vi "AlGaInPAs_v19.vi"(2 "Debug Mode":bool, 3 "Elapsed Time(s)":dbl, 4 "State":enum16{"Edit", "Start", "Run", "End", "Idle"}(ring), 5 "Argument List In":string[](array[string])) -> (0 "Status Out":string, 1 "Argument List Out":string[](array[string]))   [LabVIEW 2011]
panel:
  in  "As gas Active":bool
  in  "As gas main":T1 caption="Al" {"Flow" format="%.2f"}
  in  "As gas copy":cluster{}
  in  "P bubbler main":cluster{"Flow":dbl, "Run":bool, "Prep":bool} caption="Al" {"Flow" format="%.2f"}
  in  "P bubbler Active":bool
  in  "P gas copy":cluster{}
  in  "P gas Active":bool
  in  "P bubbler copy":cluster{}
  in  "P gas main":cluster{"Flow":dbl, "Run":bool, "Prep":bool} caption="Al" {"Flow" format="%.2f"}
  out "Al bubbler copy":cluster{}
  in  "Al Active":bool caption="Al bubbler Active"
  out "In bubbler copy":cluster{}
  in  "In bubbler Active":bool
  in  "In main":cluster{"Flow":dbl, "Run":bool, "Prep In":bool} caption="Al" {"Flow" format="%.2f"}
  in  "Ga bubbler Active":bool caption="Active"
  out "Ga bubbler copy":cluster{}
  in  "Al bubbler":T2 {"Panel"."Al Flow" format="%.2f"}
  out "prep_done":bool
  out "run started":bool
  out "first":bool=TRUE
  out "total time":dbl
  out "is OK?":bool
  in  "Prep In":bool caption="Pre-run"
  in  "prep_time":dbl
  in  "Cancel":bool
  in  "OK":bool
  out "tTotal(s) 2":dbl
  in  "Ga Tab Control":enum32{"Page 1", "Page 2", "Page 3"}(tab)
  in  "Ga main":T3 caption="Al" {"Flow" format="%.2f"}
  in  "MFC Flows":T4={"MFC2 flow"=10.0, "MFC3 flow"=100.0, "MFC1 flow"=1.0} {"MFC1 flow" format="%.4f"; "MFC3 flow" format="%.1f"; "MFC2 flow" format="%.2f"}
  in  "Ga Calculated":u16(ring)=1 caption="Calculated" items=["Ga flow", "MFC1", "MFC2", "MFC3"]
  # "Add pre-run time to run time in editor."
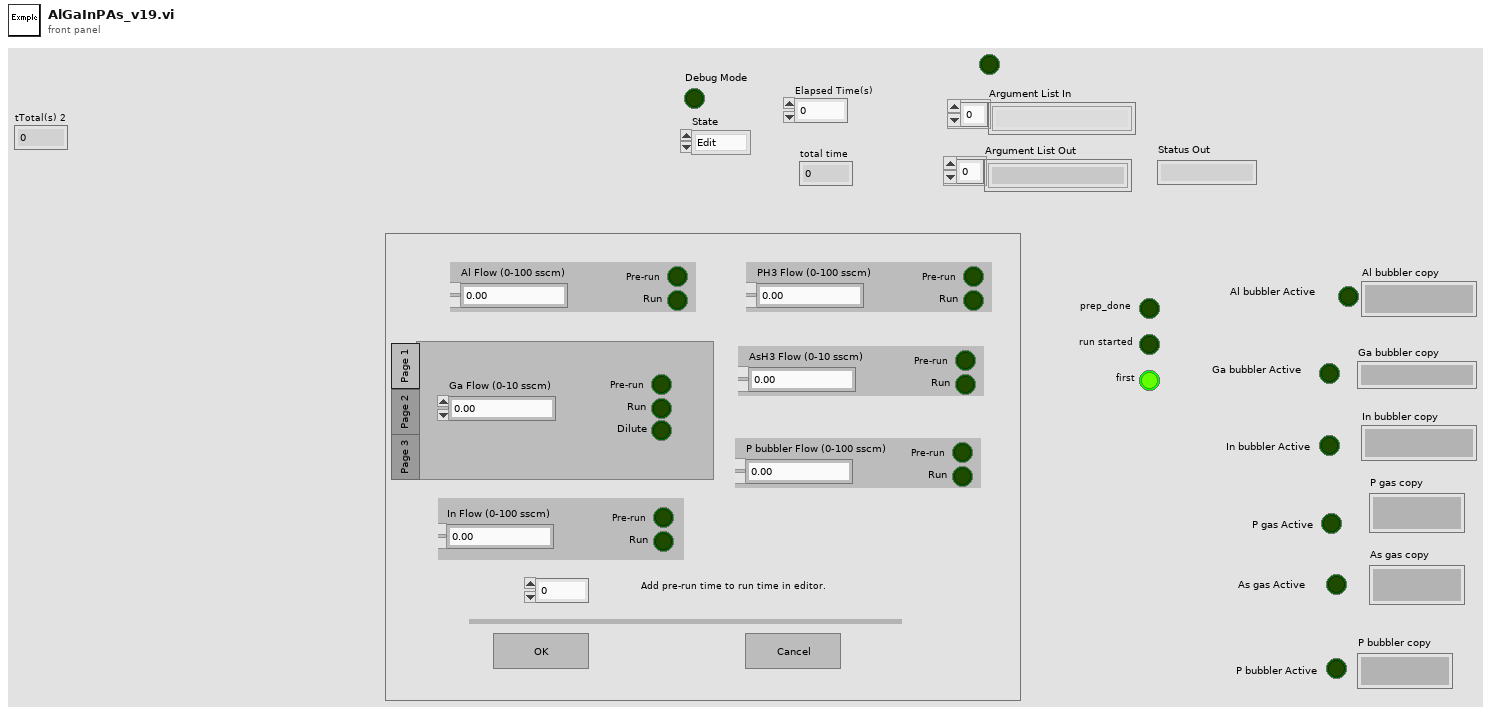
[diagram p1: front panel]
types:
  T1 = cluster{"Flow":dbl, "AsH3 Run":bool, "AsH3 Prep":bool}
  T2 = cluster{"Panel":cluster{"Al Flow":dbl, "Al Run":bool, "Prep Al":bool}}
  T3 = cluster{"Flow":dbl, "Run":bool, "Prep Ga":bool, "Dilution":bool}
  T4 = cluster{"MFC2 flow":dbl, "MFC3 flow":dbl, "MFC1 flow":dbl}
  T5 = enum16{"Discrete", "Continuous", "Instantaneous", "Finite"}
  T6 = enum32{"Invalid", "Default", "Floating", "Floating/Auto-Hide", "Modal"}
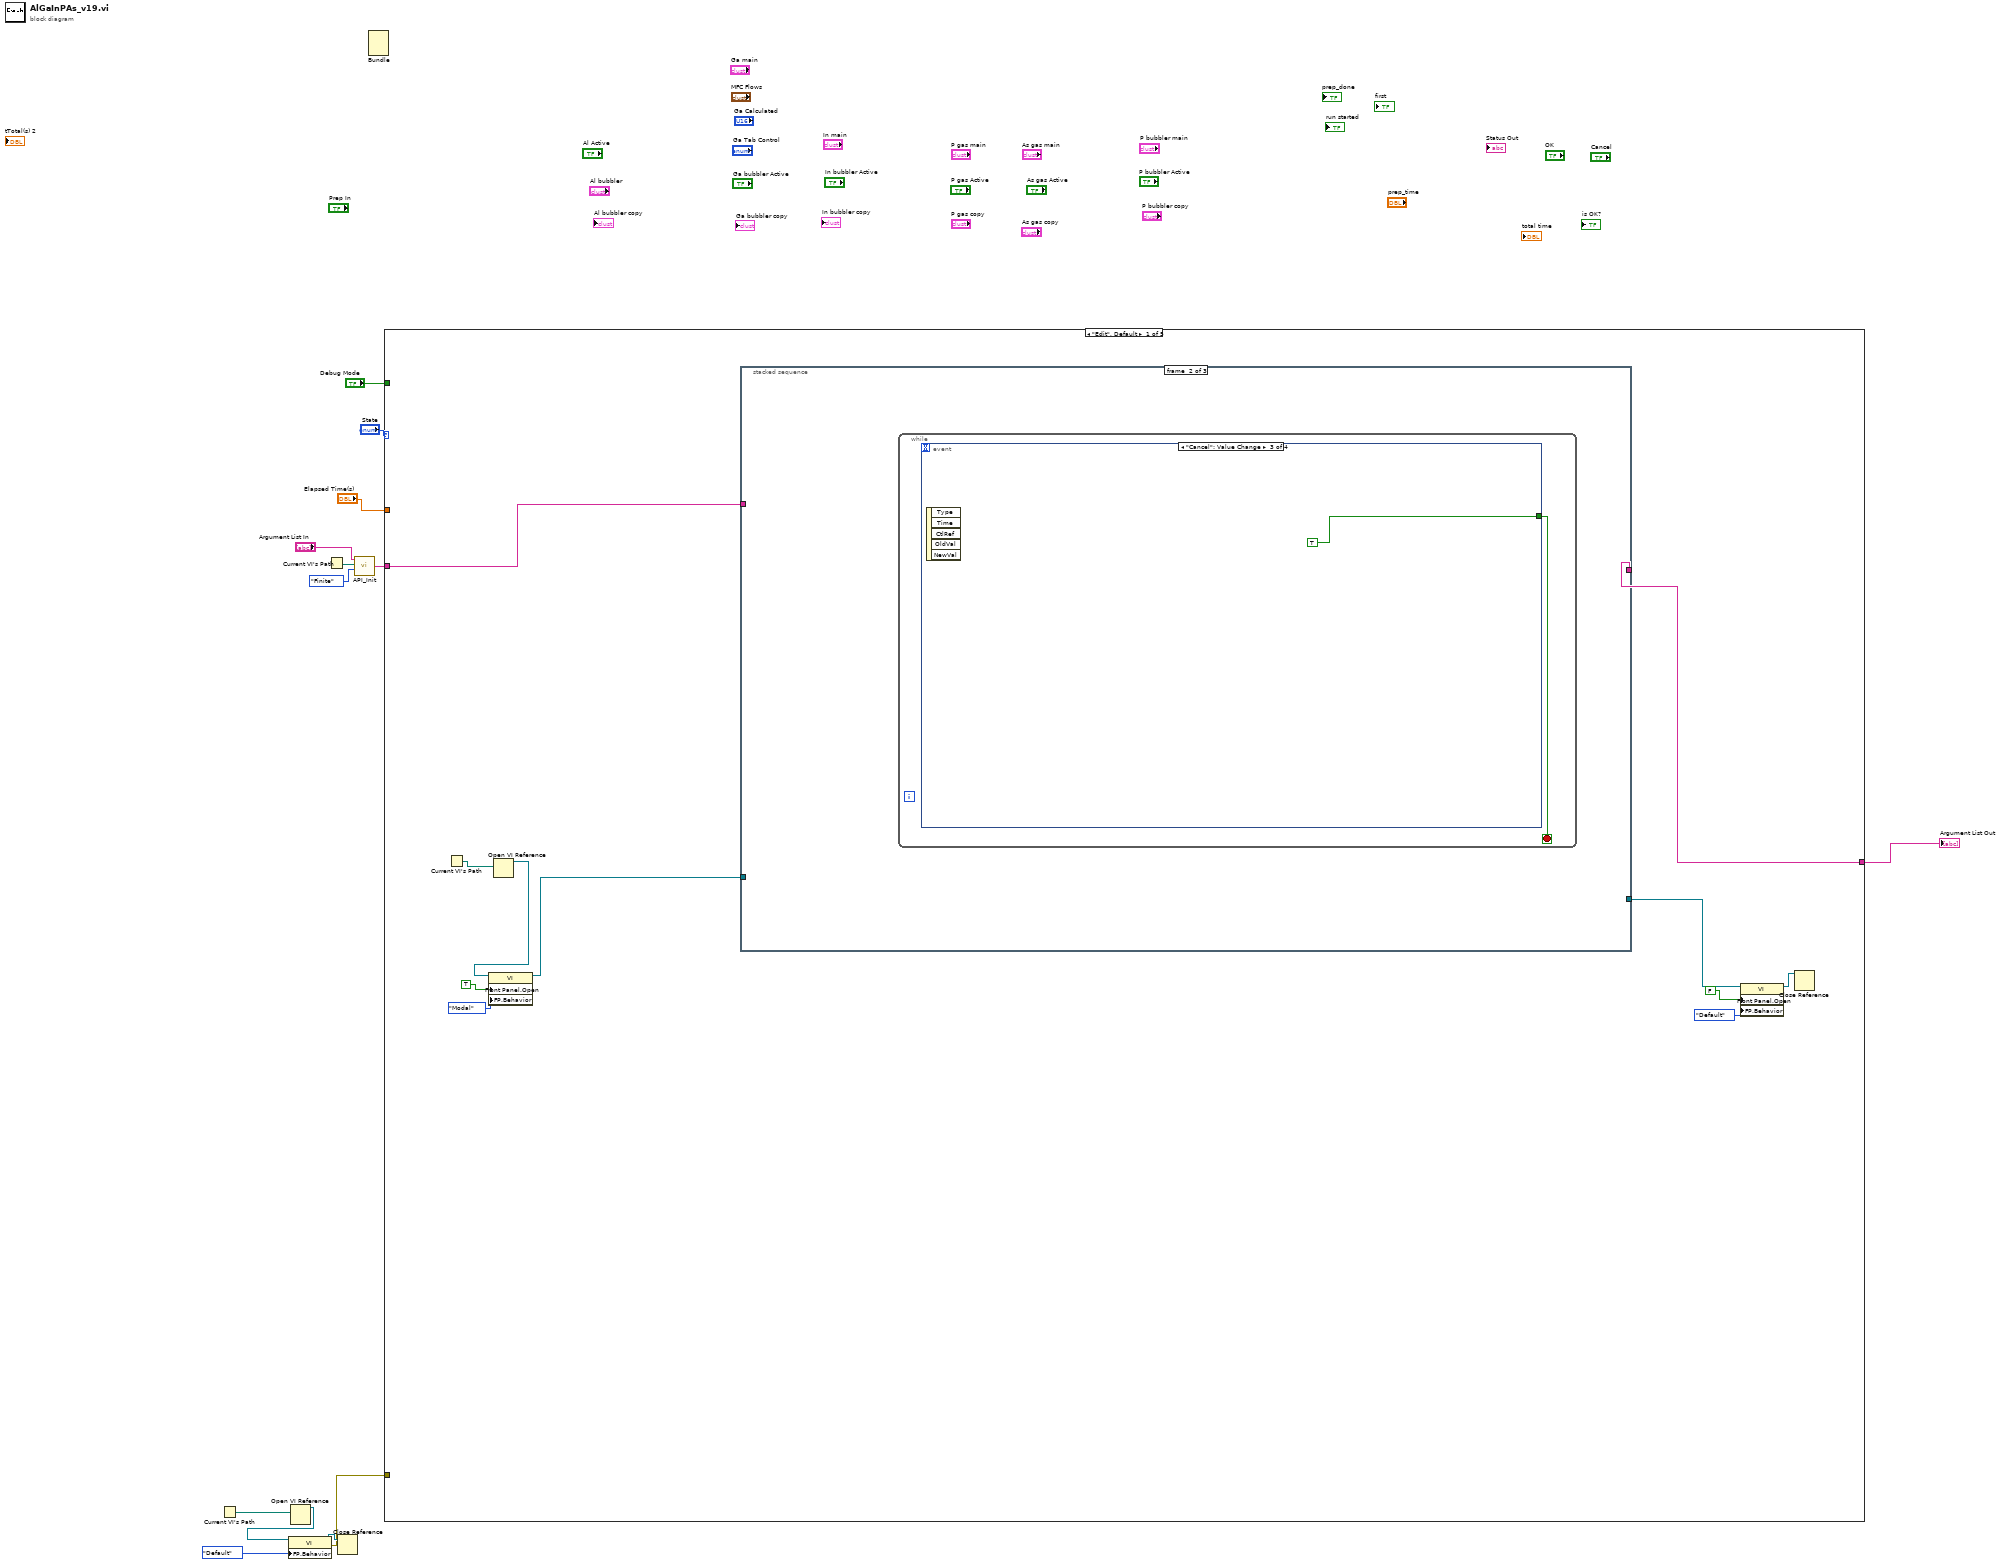
[diagram p0: block diagram]
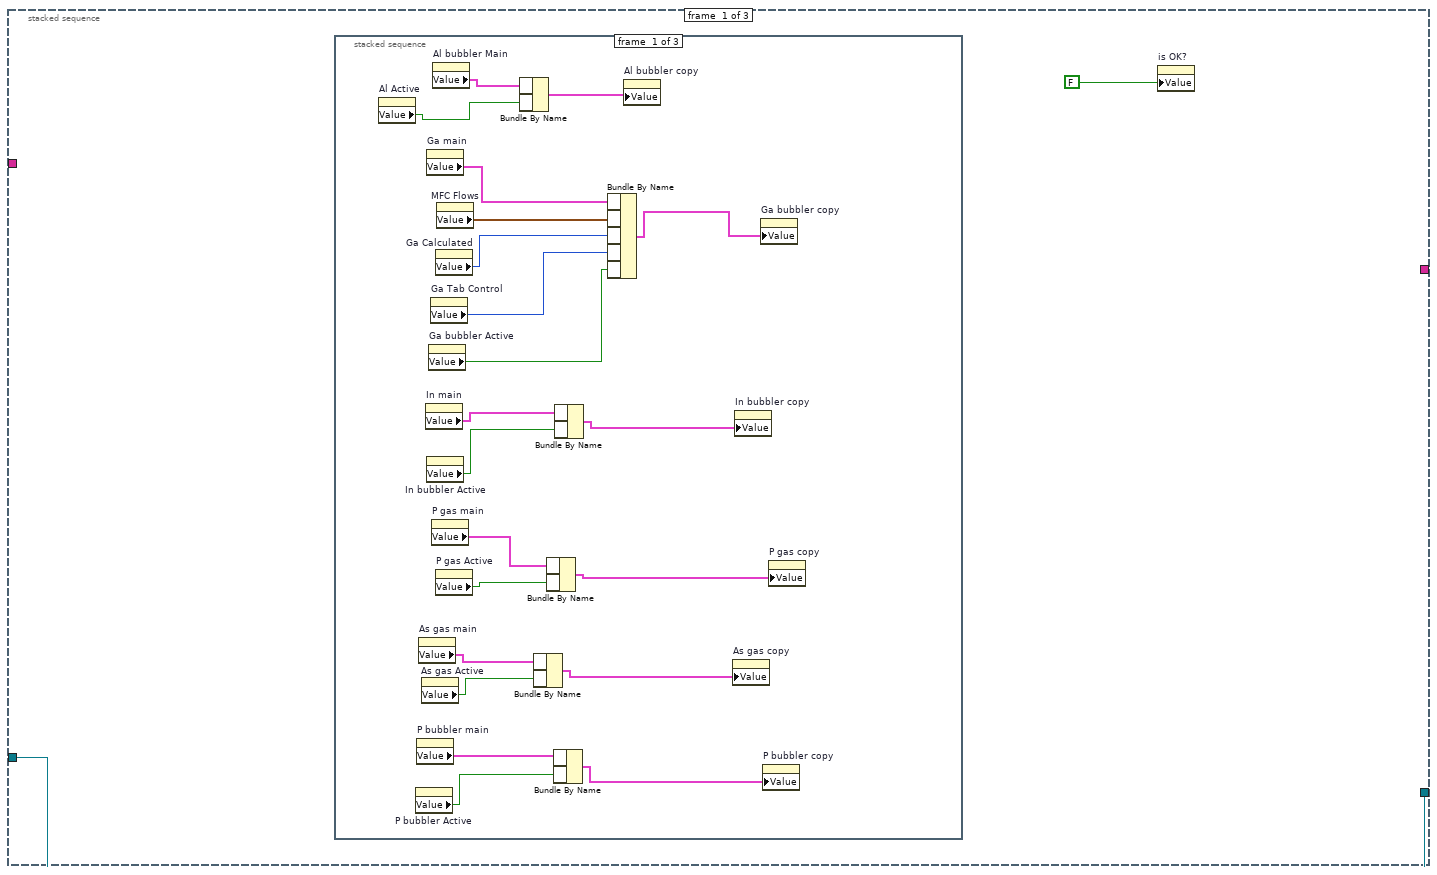
[diagram p2: hidden frame]
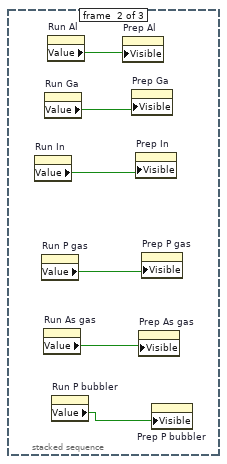
[diagram p3: hidden frame]
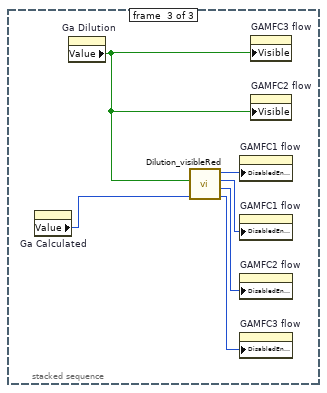
[diagram p4: hidden frame]
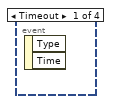
[diagram p5: hidden frame]
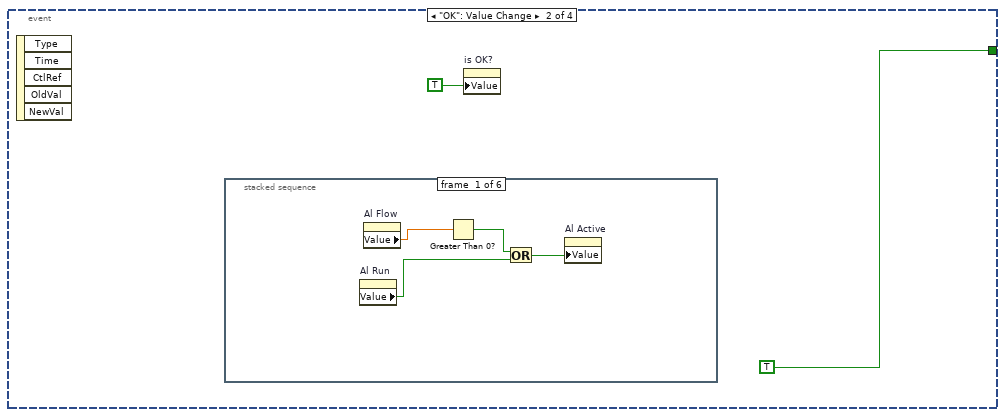
[diagram p6: hidden frame]
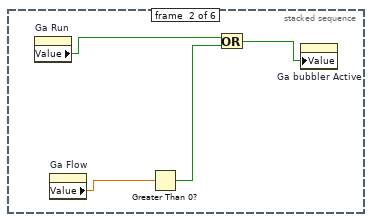
[diagram p7: hidden frame]
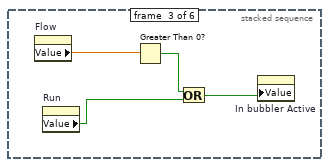
[diagram p8: hidden frame]
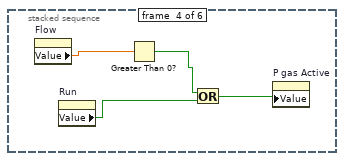
[diagram p9: hidden frame]
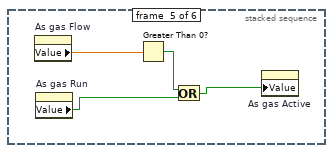
[diagram p10: hidden frame]
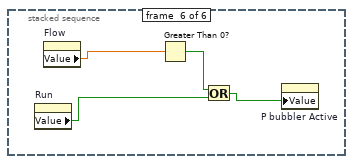
[diagram p11: hidden frame]
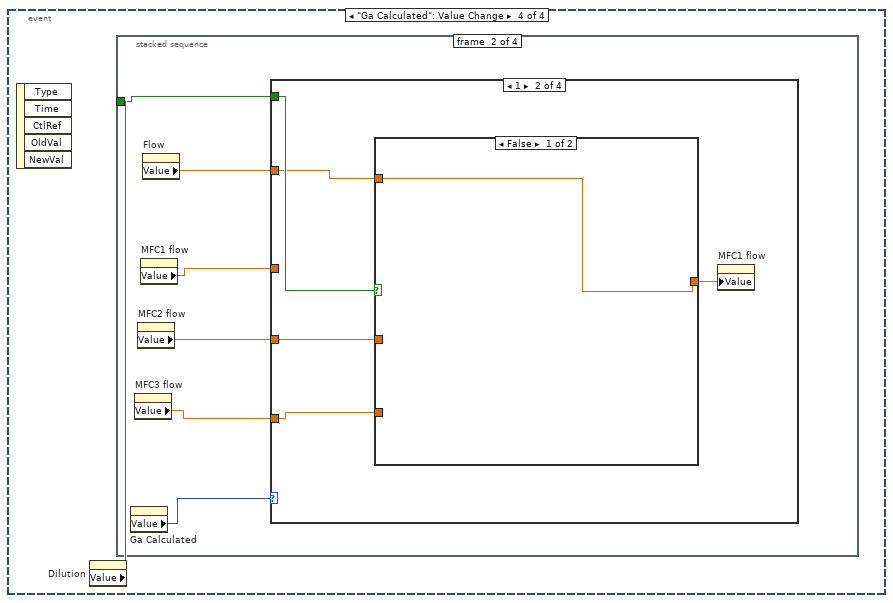
[diagram p12: hidden frame]
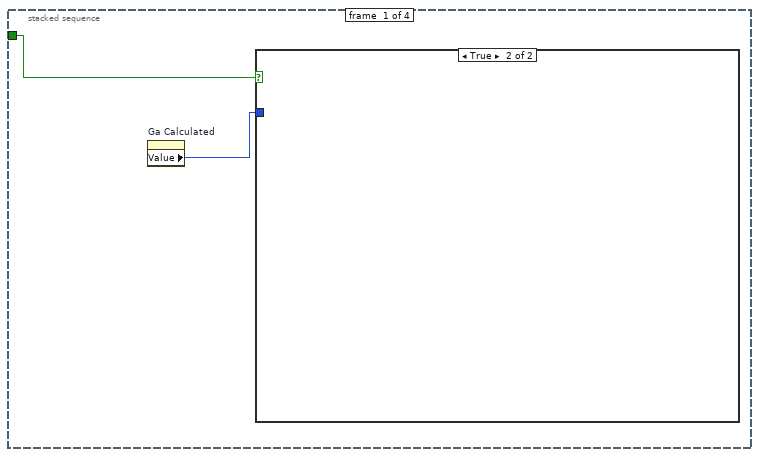
[diagram p13: hidden frame]
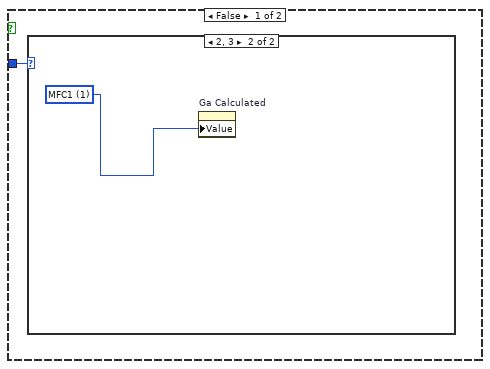
[diagram p14: hidden frame]
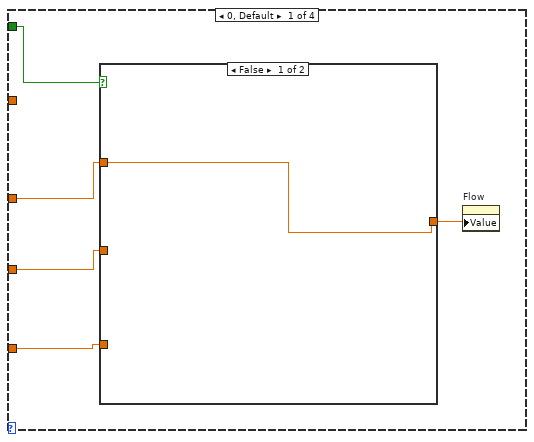
[diagram p16: hidden frame]
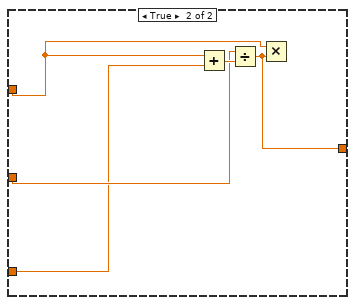
[diagram p17: hidden frame]
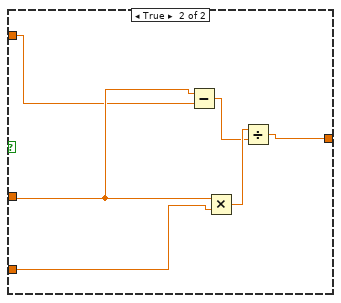
[diagram p18: hidden frame]
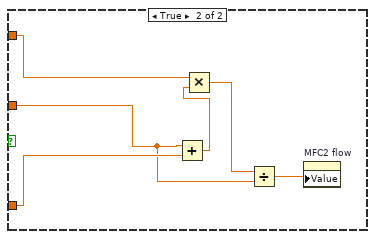
[diagram p20: hidden frame]
diagram:
  n1 = Current VI's Path() -> (path=w9:path)
  n2 = Open VI Reference(vi path=w9) -> (vi reference=w8:refnum<vi>)  [unwired: 1 in, 5 out]
  n3 = property class="VI"(reference=w8, "FP.Behavior"=T6."Default" ("Front Panel Window:Behavior")) -> (reference out=w6:refnum<vi>, error out=w5:errorcluster)  [unwired: 1 in]
  n4 = Current VI's Path() -> (path=w4:path)
  n5 = Close Reference(reference=w6) -> ()  [unwired: 1 in, 1 out]
  n6 = call "API_Init.vi"("API Mode"=T5."Finite", "VI Path"=w4, "Argument List In"="Argument List In") -> ("Argument List Out"=w1:string[])  [unwired: 1 in]
  n7 = Bundle() -> ()  [unwired: 6 in, 1 out]
  n8 = case shown="\"Edit\", Default" "State" {
    tunnel: "Debug Mode" -> [_ w159 w217 _ _]
    tunnel: "Elapsed Time(s)" -> [_ _ w218 _ _]
    tunnel: w1 -> [w15 w161 w216 w322 w323]
    tunnel: [w14 w160 w215 w322 w323] -> w10
    tunnel: w5 -> [_ _ _ _ _]
    frame "Edit", Default {
      n9 = Current VI's Path() -> (path=w20:path)
      n10 = Open VI Reference(vi path=w20) -> (vi reference=w19:refnum<vi>)  [unwired: 1 in, 5 out]
      n11 = property class="VI"(reference=w19, "Front Panel.Open"=TRUE ("Front Panel Window:Open"), "FP.Behavior"=T6."Modal" ("Front Panel Window:Behavior")) -> (reference out=w18:refnum<vi>)  [unwired: 1 in, 1 out]
      n12 = stacked-sequence {
        tunnel: w15 -> [_ _ w154]
        tunnel: w18 -> [w26 _ _]
        tunnel: [w26 _ _] -> w22
        tunnel: [_ _ w152] -> w14
        frame #0 {
          n13 = stacked-sequence {
            frame #0 {
              n14 = property on="Al Active" class="Bool (strict)"() -> ("Value"=w36:bool)  [unwired: 2 in, 2 out]
              n15 = property on="P bubbler Active" class="Bool (strict)"() -> ("Value"=w33:bool)  [unwired: 2 in, 2 out]
              n16 = property on="P bubbler main" class="Clust (strict)"() -> ("Value"=w34:cluster{"Flow":dbl, "Run":bool, "Prep":bool})  [unwired: 2 in, 2 out]
              n17 = property on="As gas main" class="Clust (strict)"() -> ("Value"=w32:T1)  [unwired: 2 in, 2 out]
              n18 = property on="As gas Active" class="Bool (strict)"() -> ("Value"=w31:bool)  [unwired: 2 in, 2 out]
              n19 = property on="In main" class="Clust (strict)"() -> ("Value"=w42:cluster{"Flow":dbl, "Run":bool, "Prep In":bool})  [unwired: 2 in, 2 out]
              n20 = property on="Ga main" class="Clust (strict)"() -> ("Value"=w39:T3)  [unwired: 2 in, 2 out]
              n21 = property on="In bubbler Active" class="Bool (strict)"() -> ("Value"=w41:bool)  [unwired: 2 in, 2 out]
              n22 = property on="Ga bubbler Active" class="Bool (strict)"() -> ("Value"=w43:bool)  [unwired: 2 in, 2 out]
              n23 = property on="Ga Tab Control" class="TabCtl (strict)"() -> ("Value"=w45:enum32{"Page 1", "Page 2", "Page 3"})  [unwired: 2 in, 2 out]
              n24 = property on="P gas main" class="Clust (strict)"() -> ("Value"=w29:cluster{"Flow":dbl, "Run":bool, "Prep":bool})  [unwired: 2 in, 2 out]
              n25 = property on="Al bubbler Main" class="Clust (strict)"() -> ("Value"=w38:T2)  [unwired: 2 in, 2 out]
              n26 = property on="Ga Calculated" class="Ring (strict)"() -> ("Value"=w46:u16)  [unwired: 2 in, 2 out]
              n27 = property on="P gas Active" class="Bool (strict)"() -> ("Value"=w28:bool)  [unwired: 2 in, 2 out]
              n28 = property on="MFC Flows" class="Clust (strict)"() -> ("Value"=w47:T4)  [unwired: 2 in, 2 out]
              n29 = Bundle By Name(w38, w36) -> (w37:cluster{})  [unwired: 1 in]
              n30 = Bundle By Name(w32, w31) -> (w30:cluster{})  [unwired: 1 in]
              n31 = Bundle By Name(w29, w28) -> (w35:cluster{})  [unwired: 1 in]
              n32 = Bundle By Name(w34, w33) -> (w27:cluster{})  [unwired: 1 in]
              n33 = Bundle By Name(w42, w41) -> (w40:cluster{})  [unwired: 1 in]
              n34 = Bundle By Name(w39, w47, w46, w45, w43) -> (w44:cluster{})  [unwired: 1 in]
              n35 = property on="Al bubbler copy" class="Clust"("Value"=w37) -> ()  [unwired: 2 in, 2 out]
              n36 = property on="As gas copy" class="Clust"("Value"=w30) -> ()  [unwired: 2 in, 2 out]
              n37 = property on="In bubbler copy" class="Clust"("Value"=w40) -> ()  [unwired: 2 in, 2 out]
              n38 = property on="Ga bubbler copy" class="Clust"("Value"=w44) -> ()  [unwired: 2 in, 2 out]
              n39 = property on="P bubbler copy" class="Clust"("Value"=w27) -> ()  [unwired: 2 in, 2 out]
              n40 = property on="P gas copy" class="Clust"("Value"=w35) -> ()  [unwired: 2 in, 2 out]
            }
            frame #1 {
              n41 = property on="Run In" class="Bool (strict)"() -> ("Value"=w52:bool)  [unwired: 2 in, 2 out]
              n42 = property on="Run P gas" class="Bool (strict)"() -> ("Value"=w50:bool)  [unwired: 2 in, 2 out]
              n43 = property on="Run As gas" class="Bool (strict)"() -> ("Value"=w49:bool)  [unwired: 2 in, 2 out]
              n44 = property on="Run Ga" class="Bool (strict)"() -> ("Value"=w51:bool)  [unwired: 2 in, 2 out]
              n45 = property on="Run Al" class="Bool (strict)"() -> ("Value"=w53:bool)  [unwired: 2 in, 2 out]
              n46 = property on="Run P bubbler" class="Bool (strict)"() -> ("Value"=w48:bool)  [unwired: 2 in, 2 out]
              n47 = property on="Prep Al" class="Bool (strict)"("Visible"=w53) -> ()  [unwired: 2 in, 2 out]
              n48 = property on="Prep Ga" class="Bool (strict)"("Visible"=w51) -> ()  [unwired: 2 in, 2 out]
              n49 = property on="Prep In" class="Bool (strict)"("Visible"=w52) -> ()  [unwired: 2 in, 2 out]
              n50 = property on="Prep As gas" class="Bool (strict)"("Visible"=w49) -> ()  [unwired: 2 in, 2 out]
              n51 = property on="Prep P gas" class="Bool (strict)"("Visible"=w50) -> ()  [unwired: 2 in, 2 out]
              n52 = property on="Prep P bubbler" class="Bool (strict)"("Visible"=w48) -> ()  [unwired: 2 in, 2 out]
            }
            frame #2 {
              n53 = property on="Ga Calculated" class="Ring (strict)"() -> ("Value"=w59:u16)  [unwired: 2 in, 2 out]
              n54 = property on="Ga Dilution" class="Bool (strict)"() -> ("Value"=w58:bool)  [unwired: 2 in, 2 out]
              n55 = call "Dilution_visibleRed.vi"("calculated"=w59, "dilution"=w58) -> ("MFC3"=w54:u16, "MFC2"=w55:u16, "MFC1"=w56:u16, "flow"=w57:u16)  [unwired: 2 in]
              n56 = property on="GAMFC1 flow" class="DigNum (strict)"("DisabledEnum"=w57) -> ()  [unwired: 2 in, 2 out]
              n57 = property on="GAMFC1 flow" class="DigNum (strict)"("DisabledEnum"=w56) -> ()  [unwired: 2 in, 2 out]
              n58 = property on="GAMFC2 flow" class="DigNum (strict)"("DisabledEnum"=w55) -> ()  [unwired: 2 in, 2 out]
              n59 = property on="GAMFC3 flow" class="DigNum (strict)"("DisabledEnum"=w54) -> ()  [unwired: 2 in, 2 out]
              n60 = property on="GAMFC3 flow" class="DigNum (strict)"("Visible"=w58) -> ()  [unwired: 2 in, 2 out]
              n61 = property on="GAMFC2 flow" class="DigNum (strict)"("Visible"=w58) -> ()  [unwired: 2 in, 2 out]
            }
          }
          n62 = property on="is OK?" class="Bool (strict)"("Value"=FALSE ("is OK?")) -> ()  [unwired: 2 in, 2 out]
        }
        frame #1 {
          n63 = while {
            stop <- w60 stop-if-true
            n64 = event shown="[2] \"Cancel\": Value Change" {
              selector: _ -> [_ _ _ _]
              dyn-events: _ -> [_ _ _ _]
              timeout: _ -> [_ _ _ _]
              tunnel: [_ TRUE TRUE _] -> w60
              event Timeout {
                n65 = event-data() -> ()  [unwired: 1 in, 2 out]
              }
              event "OK": Value Change {
                n66 = event-data() -> ()  [unwired: 1 in, 5 out]
                n67 = stacked-sequence {
                  frame #0 {
                    n68 = property on="Al Run" class="Bool (strict)"() -> ("Value"=w64:bool)  [unwired: 2 in, 2 out]
                    n69 = property on="Al Flow" class="DigNum (strict)"() -> ("Value"=w65:dbl)  [unwired: 2 in, 2 out]
                    n70 = Greater Than 0?(x=w65) -> (x > 0?=w66:bool)
                    n71 = Or(x=w66, y=w64) -> (x .or. y?=w63:bool)
                    n72 = property on="Al Active" class="Bool (strict)"("Value"=w63) -> ()  [unwired: 2 in, 2 out]
                  }
                  frame #1 {
                    n73 = property on="Ga Run" class="Bool (strict)"() -> ("Value"=w68:bool)  [unwired: 2 in, 2 out]
                    n74 = property on="Ga Flow" class="DigNum (strict)"() -> ("Value"=w67:dbl)  [unwired: 2 in, 2 out]
                    n75 = Greater Than 0?(x=w67) -> (x > 0?=w70:bool)
                    n76 = Or(x=w68, y=w70) -> (x .or. y?=w69:bool)
                    n77 = property on="Ga bubbler Active" class="Bool (strict)"("Value"=w69) -> ()  [unwired: 2 in, 2 out]
                  }
                  frame #2 {
                    n78 = property on="Flow" class="DigNum (strict)"() -> ("Value"=w73:dbl)  [unwired: 2 in, 2 out]
                    n79 = property on="Run" class="Bool (strict)"() -> ("Value"=w72:bool)  [unwired: 2 in, 2 out]
                    n80 = Greater Than 0?(x=w73) -> (x > 0?=w74:bool)
                    n81 = Or(x=w74, y=w72) -> (x .or. y?=w71:bool)
                    n82 = property on="In bubbler Active" class="Bool (strict)"("Value"=w71) -> ()  [unwired: 2 in, 2 out]
                  }
                  frame #3 {
                    n83 = property on="Flow" class="DigNum (strict)"() -> ("Value"=w77:dbl)  [unwired: 2 in, 2 out]
                    n84 = property on="Run" class="Bool (strict)"() -> ("Value"=w76:bool)  [unwired: 2 in, 2 out]
                    n85 = Greater Than 0?(x=w77) -> (x > 0?=w78:bool)
                    n86 = Or(x=w78, y=w76) -> (x .or. y?=w75:bool)
                    n87 = property on="P gas Active" class="Bool (strict)"("Value"=w75) -> ()  [unwired: 2 in, 2 out]
                  }
                  frame #4 {
                    n88 = property on="As gas Flow" class="DigNum (strict)"() -> ("Value"=w81:dbl)  [unwired: 2 in, 2 out]
                    n89 = property on="As gas Run" class="Bool (strict)"() -> ("Value"=w80:bool)  [unwired: 2 in, 2 out]
                    n90 = Greater Than 0?(x=w81) -> (x > 0?=w82:bool)
                    n91 = Or(x=w82, y=w80) -> (x .or. y?=w79:bool)
                    n92 = property on="As gas Active" class="Bool (strict)"("Value"=w79) -> ()  [unwired: 2 in, 2 out]
                  }
                  frame #5 {
                    n93 = property on="Run" class="Bool (strict)"() -> ("Value"=w84:bool)  [unwired: 2 in, 2 out]
                    n94 = property on="Flow" class="DigNum (strict)"() -> ("Value"=w85:dbl)  [unwired: 2 in, 2 out]
                    n95 = Greater Than 0?(x=w85) -> (x > 0?=w86:bool)
                    n96 = Or(x=w86, y=w84) -> (x .or. y?=w83:bool)
                    n97 = property on="P bubbler Active" class="Bool (strict)"("Value"=w83) -> ()  [unwired: 2 in, 2 out]
                  }
                }
                n98 = property on="is OK?" class="Bool (strict)"("Value"=TRUE ("is OK?")) -> ()  [unwired: 2 in, 2 out]
              }
              event "Cancel": Value Change {
                n99 = event-data() -> ()  [unwired: 1 in, 5 out]
              }
              event "Ga Calculated", "MFC Flows.MFC1 flow", "MFC Flows.MFC2 flow", "MFC Flows.MFC3 flow", "Ga main.Flow", "Ga main.Dilution": Value Change {
                n100 = event-data() -> ()  [unwired: 1 in, 5 out]
                n101 = property on="Dilution" class="Bool (strict)"() -> ("Value"=w88:bool)  [unwired: 2 in, 2 out]
                n102 = stacked-sequence {
                  tunnel: w88 -> [w89 w97 w142 w148]
                  frame #0 {
                    n103 = property on="Ga Calculated" class="Ring (strict)"() -> ("Value"=w90:u16)  [unwired: 2 in, 2 out]
                    n104 = case shown="True" w89 {
                      tunnel: w90 -> [w91 _]
                      frame False {
                        n105 = case shown="2, 3" w91 {
                          frame 0, 1, Default {
                          }
                          frame 2, 3 {
                            w92 = u16 1 items=["Ga flow", "MFC1", "MFC2", "MFC3"] ("Ga calculated")
                            n106 = property on="Ga Calculated" class="Ring (strict)"("Value"=w92) -> ()  [unwired: 2 in, 2 out]
                          }
                        }
                      }
                      frame True {
                      }
                    }
                  }
                  frame #1 {
                    n107 = property on="Ga Calculated" class="Ring (strict)"() -> ("Value"=w98:u16)  [unwired: 2 in, 2 out]
                    n108 = property on="MFC3 flow" class="DigNum (strict)"() -> ("Value"=w94:dbl)  [unwired: 2 in, 2 out]
                    n109 = property on="MFC2 flow" class="DigNum (strict)"() -> ("Value"=w95:dbl)  [unwired: 2 in, 2 out]
                    n110 = property on="MFC1 flow" class="DigNum (strict)"() -> ("Value"=w96:dbl)  [unwired: 2 in, 2 out]
                    n111 = property on="Flow" class="DigNum (strict)"() -> ("Value"=w93:dbl)  [unwired: 2 in, 2 out]
                    n112 = case shown="1" w98 {
                      tunnel: w97 -> [w103 w114 w125 w135]
                      tunnel: w96 -> [w102 _ w124 w134]
                      tunnel: w95 -> [w101 w111 _ w132]
                      tunnel: w94 -> [w100 w110 w123 _]
                      tunnel: w93 -> [_ w113 w122 w133]
                      frame 0, Default {
                        n113 = case shown="False" w103 {
                          tunnel: w102 -> [w104 w108]
                          tunnel: w101 -> [_ w107]
                          tunnel: w100 -> [_ w106]
                          tunnel: [w104 w105] -> w99
                          frame False {
                          }
                          frame True {
                            n114 = Add(x=w108, y=w106) -> (x+y=w109:dbl)
                            n115 = Divide(x=w107, y=w109) -> (x/y=w105:dbl)
                            n116 = Multiply(x=w108, y=w105) -> ()  [unwired: 1 out]
                          }
                        }
                        n117 = property on="Flow" class="DigNum (strict)"("Value"=w99) -> ()  [unwired: 2 in, 2 out]
                      }
                      frame 1 {
                        n118 = case shown="False" w114 {
                          tunnel: w113 -> [w115 w117]
                          tunnel: [w115 w116] -> w112
                          tunnel: w111 -> [_ w119]
                          tunnel: w110 -> [_ w118]
                          frame False {
                          }
                          frame True {
                            n119 = Subtract(x=w119, y=w117) -> (x-y=w120:dbl)
                            n120 = Multiply(x=w119, y=w118) -> (x*y=w121:dbl)
                            n121 = Divide(x=w121, y=w120) -> (x/y=w116:dbl)
                          }
                        }
                        n122 = property on="MFC1 flow" class="DigNum (strict)"("Value"=w112) -> ()  [unwired: 2 in, 2 out]
                      }
                      frame 2 {
                        n123 = case shown="False" w125 {
                          tunnel: w124 -> [_ w127]
                          tunnel: w123 -> [_ w129]
                          tunnel: w122 -> [_ w128]
                          frame False {
                          }
                          frame True {
                            n124 = Add(x=w127, y=w129) -> (x+y=w131:dbl)
                            n125 = Multiply(x=w128, y=w131) -> (x*y=w130:dbl)
                            n126 = Divide(x=w130, y=w127) -> (x/y=w126:dbl)
                            n127 = property on="MFC2 flow" class="DigNum (strict)"("Value"=w126) -> ()  [unwired: 2 in, 2 out]
                          }
                        }
                      }
                      frame 3 {
                        n128 = case shown="False" w135 {
                          tunnel: w134 -> [_ w139]
                          tunnel: w133 -> [_ w138]
                          tunnel: w132 -> [_ w137]
                          frame False {
                          }
                          frame True {
                            n129 = Subtract(x=w137, y=w138) -> (x-y=w140:dbl)
                            n130 = Divide(x=w139, y=w138) -> (x/y=w141:dbl)
                            n131 = Multiply(x=w141, y=w140) -> (x*y=w136:dbl)
                            n132 = property on="MFC3 flow" class="DigNum (strict)"("Value"=w136) -> ()  [unwired: 2 in, 2 out]
                          }
                        }
                      }
                    }
                  }
                  frame #2 {
                    n133 = property on="Ga Calculated" class="Ring (strict)"() -> ("Value"=w147:u16)  [unwired: 2 in, 2 out]
                    n134 = call "Dilution_visibleRed.vi"("calculated"=w147, "dilution"=w142) -> ("MFC3"=w143:u16, "MFC2"=w144:u16, "MFC1"=w145:u16, "flow"=w146:u16)  [unwired: 2 in]
                    n135 = property on="MFC3 flow" class="DigNum (strict)"("Visible"=w142) -> ()  [unwired: 2 in, 2 out]
                    n136 = property on="Flow" class="DigNum (strict)"("DisabledEnum"=w146) -> ()  [unwired: 2 in, 2 out]
                    n137 = property on="MFC3 flow" class="DigNum (strict)"("DisabledEnum"=w143) -> ()  [unwired: 2 in, 2 out]
                    n138 = property on="MFC2 flow" class="DigNum (strict)"("Visible"=w142) -> ()  [unwired: 2 in, 2 out]
                    n139 = property on="MFC2 flow" class="DigNum (strict)"("DisabledEnum"=w144) -> ()  [unwired: 2 in, 2 out]
                    n140 = property on="MFC1 flow" class="DigNum (strict)"("DisabledEnum"=w145) -> ()  [unwired: 2 in, 2 out]
                  }
                  frame #3 {
                    n141 = case shown="True" w148 {
                      frame False {
                        n142 = property on="Ga Calculated" class="Ring (strict)"("Disabled Items []"=i32[] [2, 3]) -> ()  [unwired: 2 in, 2 out]
                      }
                      frame True {
                        n143 = property on="Ga Calculated" class="Ring (strict)"("Disabled Items []"=i32[] []) -> ()  [unwired: 2 in, 2 out]
                      }
                    }
                  }
                }
              }
            }
          }
        }
        frame #2 {
          n144 = property on="is OK?" class="Bool (strict)"() -> ("Value"=w151:bool)  [unwired: 2 in, 2 out]
          n145 = case shown="True" w151 {
            tunnel: w154 -> [w157 w158]
            tunnel: [w157 w158] -> w153
            frame False {
            }
            frame True {
            }
          }
          n146 = Not(x=w151) -> (.not. x?=w156:bool)
          n147 = Current VI's Path() -> (path=w155:path)
          n148 = call "API_Edit.vi"("Cancel"=w156, "OK"=w151, "VI Path"=w155, "Argument List In"=w153) -> ("Argument List Out"=w152:string[])
        }
      }
      n149 = property class="VI"(reference=w22, "Front Panel.Open"=FALSE ("Front Panel Window:Open"), "FP.Behavior"=T6."Default" ("Front Panel Window:Behavior")) -> (reference out=w23:refnum<vi>)  [unwired: 1 in, 1 out]
      n150 = Close Reference(reference=w23) -> ()  [unwired: 1 in, 1 out]
    }
    frame "Start" {
      n151 = call "Set_Argument.vi"("Enable"=FALSE, "Argument"="run_started", "Argument List In"=w161) -> ("Argument List Out"=w160:string[])
      n152 = case shown="False" w159 {
        frame False {
          n153 = stacked-sequence {
            frame #0 {
              n154 = property on="Al Active" class="Bool (strict)"() -> ("Value"=w164:bool)  [unwired: 2 in, 2 out]
              n155 = case shown="False" w164 {
                frame False {
                  w165 = FALSE ("Al Active")
                  n156 = call "set_Al.vi"("ALMFC1"=0.0 ("Aluminum Flow"), "Remote"=w165, "Run"=w165, "Bubbler In"=w165, "Active"=w165) -> ()  [unwired: 5 out]
                }
                frame True {
                  w171 = TRUE ("Al Active")
                  n157 = property on="Al Run" class="Bool (strict)"() -> ("Value"=w167:bool)  [unwired: 2 in, 2 out]
                  n158 = property on="Prep Al" class="Bool (strict)"() -> ("Value"=w168:bool)  [unwired: 2 in, 2 out]
                  n159 = And(x=w168, y=w167) -> (x .and. y?=w170:bool)
                  n160 = property on="Al Flow" class="DigNum (strict)"() -> ("Value"=w169:dbl)  [unwired: 2 in, 2 out]
                  n161 = call "set_Al.vi"("ALMFC1"=w169, "Run"=w170, "Bubbler In"=w171, "Active"=w171) -> ()  [unwired: 1 in, 5 out]
                }
              }
            }
            frame #1 {
              n162 = property on="Ga bubbler Active" class="Bool (strict)"() -> ("Value"=w172:bool)  [unwired: 2 in, 2 out]
              n163 = case shown="True" w172 {
                frame False {
                  w174 = FALSE ("Ga Active")
                  w173 = 0.0 ("Ga Flow 1")
                  n164 = call "set_Ga.vi"("Active"=w174, "GAMFC3"=w173, "GAMFC2"=w173, "GAMFC1"=w173, "Bubbler In"=w174, "H2 Dilute"=w174, "Run"=w174, "Remote"=w174) -> ()  [unwired: 8 out]
                }
                frame True {
                  w181 = TRUE ("Ga Active")
                  n165 = property on="Prep Ga" class="Bool (strict)"() -> ("Value"=w178:bool)  [unwired: 2 in, 2 out]
                  n166 = property on="Dilution" class="Bool (strict)"() -> ("Value"=w180:bool)  [unwired: 2 in, 2 out]
                  n167 = property on="MFC1 flow" class="DigNum (strict)"() -> ("Value"=w177:dbl)  [unwired: 2 in, 2 out]
                  n168 = property on="Run" class="Bool (strict)"() -> ("Value"=w179:bool)  [unwired: 2 in, 2 out]
                  n169 = And(x=w178, y=w179) -> (x .and. y?=w182:bool)
                  n170 = property on="MFC2 flow" class="DigNum (strict)"() -> ("Value"=w176:dbl)  [unwired: 2 in, 2 out]
                  n171 = property on="MFC3 flow" class="DigNum (strict)"() -> ("Value"=w175:dbl)  [unwired: 2 in, 2 out]
                  n172 = call "set_Ga.vi"("Active"=w181, "GAMFC3"=w175, "GAMFC2"=w176, "GAMFC1"=w177, "Bubbler In"=w181, "H2 Dilute"=w180, "Run"=w182, "Remote"=w181) -> ()  [unwired: 8 in]
                }
              }
            }
            frame #2 {
              n173 = property on="In bubbler Active" class="Bool (strict)"() -> ("Value"=w183:bool)  [unwired: 2 in, 2 out]
              n174 = case shown="False" w183 {
                frame False {
                  w185 = FALSE ("In Remote")
                  n175 = call "set_In.vi"("INMFC1"=0.0 ("Indium Flow"), "Remote"=w185, "Run"=w185, "Bubbler In"=w185, "Active"=w185) -> ()  [unwired: 5 out]
                }
                frame True {
                  w190 = TRUE ("In Run")
                  n176 = property on="Run" class="Bool (strict)"() -> ("Value"=w187:bool)  [unwired: 2 in, 2 out]
                  n177 = property on="Prep In" class="Bool (strict)"() -> ("Value"=w188:bool)  [unwired: 2 in, 2 out]
                  n178 = And(x=w187, y=w188) -> (x .and. y?=w189:bool)
                  n179 = property on="Flow" class="DigNum (strict)"() -> ("Value"=w186:dbl)  [unwired: 2 in, 2 out]
                  n180 = call "set_In.vi"("INMFC1"=w186, "Run"=w189, "Bubbler In"=w190, "Active"=w190) -> ()  [unwired: 1 in, 5 out]
                }
              }
            }
            frame #3 {
              n181 = property on="P gas Active" class="Bool (strict)"() -> ("Value"=w191:bool)  [unwired: 2 in, 2 out]
              n182 = case shown="False" w191 {
                frame False {
                  w192 = FALSE ("P_Gas Active")
                  n183 = call "set_P_gas.vi"("Run"=w192, "Gas In"=w192, "Active"=w192, "P_Gas Remote"=w192, "H2 Flush"=w192, "P_Gas Flow"=0.0) -> ()
                }
                frame True {
                  w198 = TRUE ("P_Gas Active")
                  n184 = property on="Flow" class="DigNum (strict)"() -> ("Value"=w196:dbl)  [unwired: 2 in, 2 out]
                  n185 = property on="Prep" class="Bool (strict)"() -> ("Value"=w195:bool)  [unwired: 2 in, 2 out]
                  n186 = property on="Run" class="Bool (strict)"() -> ("Value"=w194:bool)  [unwired: 2 in, 2 out]
                  n187 = And(x=w195, y=w194) -> (x .and. y?=w197:bool)
                  n188 = call "set_P_gas.vi"("Active"=w198, "P_Gas Remote"=w197, "H2 Flush"=w198, "P_Gas Flow"=w196) -> ()  [unwired: 2 in]
                }
              }
            }
            frame #4 {
              n189 = property on="As gas Active" class="Bool (strict)"() -> ("Value"=w199:bool)  [unwired: 2 in, 2 out]
              n190 = case shown="False" w199 {
                frame False {
                  w200 = FALSE ("As_Gas Active")
                  n191 = call "set_As_gas.vi"("Active"=w200, "As_Gas Flow"=0.0, "Gas In"=w200, "H2 Flush"=w200, "Run"=w200, "Remote"=w200) -> ()  [unwired: 10 in]
                }
                frame True {
                  w206 = TRUE ("As_Gas Active")
                  n192 = property on="AsH3 Run" class="Bool (strict)"() -> ("Value"=w202:bool)  [unwired: 2 in, 2 out]
                  n193 = property on="AsH3 Prep" class="Bool (strict)"() -> ("Value"=w203:bool)  [unwired: 2 in, 2 out]
                  n194 = And(x=w203, y=w202) -> (x .and. y?=w205:bool)
                  n195 = property on="Flow" class="DigNum (strict)"() -> ("Value"=w204:dbl)  [unwired: 2 in, 2 out]
                  n196 = call "set_As_gas.vi"("Active"=w206, "As_Gas Flow"=w204, "Gas In"=w206, "Run"=w205) -> ()  [unwired: 12 in]
                }
              }
            }
            frame #5 {
              n197 = property on="P bubbler Active" class="Bool (strict)"() -> ("Value"=w207:bool)  [unwired: 2 in, 2 out]
              n198 = case shown="False" w207 {
                frame False {
                  w208 = FALSE ("As_Gas Active")
                  n199 = call "set_P_Liq.vi"("flow 1"=0.0 ("As_Gas Flow"), "Remote"=w208, "Run"=w208, "Bubbler In"=w208, "Active"=w208) -> ()  [unwired: 5 in]
                }
                frame True {
                  w214 = TRUE ("As_Gas Active")
                  n200 = property on="Run" class="Bool (strict)"() -> ("Value"=w210:bool)  [unwired: 2 in, 2 out]
                  n201 = property on="Prep" class="Bool (strict)"() -> ("Value"=w211:bool)  [unwired: 2 in, 2 out]
                  n202 = And(x=w211, y=w210) -> (x .and. y?=w213:bool)
                  n203 = property on="Flow" class="DigNum (strict)"() -> ("Value"=w212:dbl)  [unwired: 2 in, 2 out]
                  n204 = call "set_P_Liq.vi"("flow 1"=w212, "Run"=w213, "Bubbler In"=w214, "Active"=w214) -> ()  [unwired: 6 in]
                }
              }
            }
          }
        }
        frame True {
        }
      }
    }
    frame "Run" {
      n205 = stacked-sequence {
        tunnel: w218 -> [_ w223 _ _]
        tunnel: w216 -> [w220 _ _ w275]
        tunnel: w217 -> [_ _ _ w274]
        tunnel: [_ _ _ w268] -> w215
        frame #0 {
          n206 = call "Get_Argument.vi"("Argument"="run_started", "Argument List"=w220) -> ("Enabled"=w219:bool)
          n207 = local write "run started"(w219) -> ()
        }
        frame #1 {
          n208 = property on="prep_time" class="DigNum (strict)"() -> ("Value"=w224:dbl)  [unwired: 2 in, 2 out]
          n209 = Greater Or Equal?(x=w223, y=w224) -> (x >= y?=w222:bool)
          n210 = local write "prep_done"(w222) -> ()
        }
        frame #2 {
          n211 = local read "run started"() -> (w226:bool)
          n212 = Not(x=w226) -> (.not. x?=w225:bool)
          n213 = stacked-sequence {
            tunnel: w225 -> [w228 w231 w237 w243 w250 w256 w262]
            frame #0 {
              n214 = case shown="True" w228 {
                tunnel: ["run: " "pre-run: "] -> w227
                frame False {
                }
                frame True {
                }
              }
              n215 = property on="Status Out" class="Str"("Value"=w227) -> ()  [unwired: 2 in, 2 out]
            }
            frame #1 {
              n216 = property on="Status Out" class="Str"() -> ("Value"=w236:string)  [unwired: 2 in, 2 out]
              n217 = call "flow_strings.vi"("string in"=w236, "is first in?"=TRUE, "name"="Al", "is prep?"=w231) -> ("string out"=w235:string, "is first out?"=w234:bool)  [unwired: 3 in]
              n218 = property on="Status Out" class="Str"("Value"=w235) -> ()  [unwired: 2 in, 2 out]
              n219 = property on="first" class="Bool (strict)"("Value"=w234) -> ()  [unwired: 2 in, 2 out]
            }
            frame #2 {
              n220 = property on="first" class="Bool (strict)"() -> ("Value"=w239:bool)  [unwired: 2 in, 2 out]
              n221 = property on="Status Out" class="Str"() -> ("Value"=w241:string)  [unwired: 2 in, 2 out]
              n222 = call "flow_strings.vi"("string in"=w241, "is first in?"=w239, "name"="Ga", "is prep?"=w237) -> ("string out"=w242:string, "is first out?"=w238:bool)  [unwired: 3 in]
              n223 = property on="Status Out" class="Str"("Value"=w242) -> ()  [unwired: 2 in, 2 out]
              n224 = property on="first" class="Bool (strict)"("Value"=w238) -> ()  [unwired: 2 in, 2 out]
            }
            frame #3 {
              n225 = property on="first" class="Bool (strict)"() -> ("Value"=w247:bool)  [unwired: 2 in, 2 out]
              n226 = property on="Status Out" class="Str"() -> ("Value"=w249:string)  [unwired: 2 in, 2 out]
              n227 = property on="Prep In" class="Bool (strict)"() -> ("Value"=w244:bool)  [unwired: 2 in, 2 out]
              n228 = call "flow_strings.vi"("string in"=w249, "is first in?"=w247, "name"="In", "prep source?"=w244, "is prep?"=w243) -> ("string out"=w246:string, "is first out?"=w245:bool)  [unwired: 2 in]
              n229 = property on="Status Out" class="Str"("Value"=w246) -> ()  [unwired: 2 in, 2 out]
              n230 = property on="first" class="Bool (strict)"("Value"=w245) -> ()  [unwired: 2 in, 2 out]
            }
            frame #4 {
              n231 = property on="first" class="Bool (strict)"() -> ("Value"=w252:bool)  [unwired: 2 in, 2 out]
              n232 = property on="Status Out" class="Str"() -> ("Value"=w254:string)  [unwired: 2 in, 2 out]
              n233 = call "flow_strings.vi"("string in"=w254, "is first in?"=w252, "name"="PH3", "is prep?"=w250) -> ("string out"=w253:string, "is first out?"=w251:bool)  [unwired: 3 in]
              n234 = property on="Status Out" class="Str"("Value"=w253) -> ()  [unwired: 2 in, 2 out]
              n235 = property on="first" class="Bool (strict)"("Value"=w251) -> ()  [unwired: 2 in, 2 out]
            }
            frame #5 {
              n236 = property on="first" class="Bool (strict)"() -> ("Value"=w258:bool)  [unwired: 2 in, 2 out]
              n237 = property on="Status Out" class="Str"() -> ("Value"=w260:string)  [unwired: 2 in, 2 out]
              n238 = call "flow_strings.vi"("string in"=w260, "is first in?"=w258, "name"="AsH3", "is prep?"=w256) -> ("string out"=w257:string, "is first out?"=w259:bool)  [unwired: 3 in]
              n239 = property on="Status Out" class="Str"("Value"=w257) -> ()  [unwired: 2 in, 2 out]
              n240 = property on="first" class="Bool (strict)"("Value"=w259) -> ()  [unwired: 2 in, 2 out]
            }
            frame #6 {
              n241 = property on="first" class="Bool (strict)"() -> ("Value"=w265:bool)  [unwired: 2 in, 2 out]
              n242 = property on="Status Out" class="Str"() -> ("Value"=w267:string)  [unwired: 2 in, 2 out]
              n243 = call "flow_strings.vi"("string in"=w267, "is first in?"=w265, "name"="P liq", "is prep?"=w262) -> ("string out"=w264:string, "is first out?"=w263:bool)  [unwired: 3 in]
              n244 = property on="Status Out" class="Str"("Value"=w264) -> ()  [unwired: 2 in, 2 out]
              n245 = property on="first" class="Bool (strict)"("Value"=w263) -> ()  [unwired: 2 in, 2 out]
            }
          }
        }
        frame #3 {
          n246 = local read "prep_done"() -> (w272:bool)
          n247 = local read "run started"() -> (w271:bool)
          n248 = Not(x=w272) -> (.not. x?=w270:bool)
          n249 = Or(x=w270, y=w271) -> (x .or. y?=w269:bool)
          n250 = Or(x=w274, y=w269) -> (x .or. y?=w273:bool)
          n251 = case shown="False" w273 {
            tunnel: w275 -> [w277 _]
            tunnel: [w276 _] -> w268
            frame False {
              n252 = stacked-sequence {
                tunnel: [_ _ _ _ _ _ w319] -> w276
                tunnel: w277 -> [_ _ _ _ _ _ w318]
                frame #0 {
                  n253 = property on="Al Active" class="Bool (strict)"() -> ("Value"=w278:bool)  [unwired: 2 in, 2 out]
                  n254 = case shown="True" w278 {
                    frame False {
                      w279 = FALSE ("Al Active")
                      n255 = call "set_Al.vi"("ALMFC1"=0.0 ("Aluminum Flow"), "Remote"=w279, "Run"=w279, "Bubbler In"=w279, "Active"=w279) -> ()  [unwired: 5 out]
                    }
                    frame True {
                      w283 = TRUE ("Al Active")
                      n256 = property on="Al Flow" class="DigNum (strict)"() -> ("Value"=w282:dbl)  [unwired: 2 in, 2 out]
                      n257 = property on="Al Run" class="Bool (strict)"() -> ("Value"=w281:bool)  [unwired: 2 in, 2 out]
                      n258 = call "set_Al.vi"("ALMFC1"=w282, "Run"=w281, "Bubbler In"=w283, "Active"=w283) -> ()  [unwired: 1 in, 5 out]
                    }
                  }
                }
                frame #1 {
                  n259 = property on="Ga bubbler Active" class="Bool (strict)"() -> ("Value"=w284:bool)  [unwired: 2 in, 2 out]
                  n260 = case shown="False" w284 {
                    frame False {
                      w286 = FALSE ("Ga Active")
                      w285 = 0.0 ("Ga Flow 1")
                      n261 = call "set_Ga.vi"("Active"=w286, "GAMFC3"=w285, "GAMFC2"=w285, "GAMFC1"=w285, "Bubbler In"=w286, "H2 Dilute"=w286, "Run"=w286, "Remote"=w286) -> ()  [unwired: 8 out]
                    }
                    frame True {
                      w292 = TRUE ("Ga Active")
                      n262 = property on="MFC2 flow" class="DigNum (strict)"() -> ("Value"=w288:dbl)  [unwired: 2 in, 2 out]
                      n263 = property on="MFC3 flow" class="DigNum (strict)"() -> ("Value"=w287:dbl)  [unwired: 2 in, 2 out]
                      n264 = property on="Run" class="Bool (strict)"() -> ("Value"=w291:bool)  [unwired: 2 in, 2 out]
                      n265 = property on="MFC1 flow" class="DigNum (strict)"() -> ("Value"=w289:dbl)  [unwired: 2 in, 2 out]
                      n266 = property on="Dilution" class="Bool (strict)"() -> ("Value"=w290:bool)  [unwired: 2 in, 2 out]
                      n267 = call "set_Ga.vi"("Active"=w292, "GAMFC3"=w287, "GAMFC2"=w288, "GAMFC1"=w289, "Bubbler In"=w292, "H2 Dilute"=w290, "Run"=w291, "Remote"=w292) -> ()  [unwired: 8 in]
                    }
                  }
                }
                frame #2 {
                  n268 = property on="In bubbler Active" class="Bool (strict)"() -> ("Value"=w293:bool)  [unwired: 2 in, 2 out]
                  n269 = case shown="True" w293 {
                    frame False {
                      w295 = FALSE ("In Remote")
                      n270 = call "set_In.vi"("INMFC1"=0.0 ("Indium Flow"), "Remote"=w295, "Run"=w295, "Bubbler In"=w295, "Active"=w295) -> ()  [unwired: 5 out]
                    }
                    frame True {
                      w298 = TRUE ("In Run")
                      n271 = property on="Run" class="Bool (strict)"() -> ("Value"=w296:bool)  [unwired: 2 in, 2 out]
                      n272 = property on="In Flow" class="DigNum (strict)"() -> ("Value"=w297:dbl)  [unwired: 2 in, 2 out]
                      n273 = call "set_In.vi"("INMFC1"=w297, "Run"=w296, "Bubbler In"=w298, "Active"=w298) -> ()  [unwired: 1 in, 5 out]
                    }
                  }
                }
                frame #3 {
                  n274 = property on="P gas Active" class="Bool (strict)"() -> ("Value"=w299:bool)  [unwired: 2 in, 2 out]
                  n275 = case shown="False" w299 {
                    frame False {
                      w300 = FALSE ("P_Gas Active")
                      n276 = call "set_P_gas.vi"("Run"=w300, "Gas In"=w300, "Active"=w300, "P_Gas Remote"=w300, "H2 Flush"=w300, "P_Gas Flow"=0.0) -> ()
                    }
                    frame True {
                      n277 = property on="Run" class="Bool (strict)"() -> ("Value"=w303:bool)  [unwired: 2 in, 2 out]
                      n278 = property on="Flow" class="DigNum (strict)"() -> ("Value"=w304:dbl)  [unwired: 2 in, 2 out]
                      n279 = call "set_P_gas.vi"("Run"=w303, "Gas In"=TRUE, "Active"=TRUE ("P_Gas Active"), "P_Gas Flow"=w304) -> ()  [unwired: 2 in]
                    }
                  }
                }
                frame #4 {
                  n280 = property on="As gas Active" class="Bool (strict)"() -> ("Value"=w306:bool)  [unwired: 2 in, 2 out]
                  n281 = case shown="True" w306 {
                    frame False {
                      w307 = FALSE ("As_Gas Active")
                      n282 = call "set_As_gas.vi"("Active"=w307, "As_Gas Flow"=0.0, "Gas In"=w307, "H2 Flush"=w307, "Run"=w307, "Remote"=w307) -> ()  [unwired: 10 in]
                    }
                    frame True {
                      w311 = TRUE ("As_Gas Active")
                      n283 = property on="AsH3 Run" class="Bool (strict)"() -> ("Value"=w310:bool)  [unwired: 2 in, 2 out]
                      n284 = property on="Flow" class="DigNum (strict)"() -> ("Value"=w309:dbl)  [unwired: 2 in, 2 out]
                      n285 = call "set_As_gas.vi"("Active"=w311, "As_Gas Flow"=w309, "Gas In"=w311, "Run"=w310) -> ()  [unwired: 12 in]
                    }
                  }
                }
                frame #5 {
                  n286 = property on="P bubbler Active" class="Bool (strict)"() -> ("Value"=w312:bool)  [unwired: 2 in, 2 out]
                  n287 = case shown="True" w312 {
                    frame False {
                      w314 = FALSE ("In Remote")
                      n288 = call "set_P_Liq.vi"("flow 1"=0.0 ("Indium Flow"), "Remote"=w314, "Run"=w314, "Bubbler In"=w314, "Active"=w314) -> ()  [unwired: 5 in]
                    }
                    frame True {
                      w317 = TRUE ("In Run")
                      n289 = property on="Flow" class="DigNum (strict)"() -> ("Value"=w316:dbl)  [unwired: 2 in, 2 out]
                      n290 = property on="Run" class="Bool (strict)"() -> ("Value"=w315:bool)  [unwired: 2 in, 2 out]
                      n291 = call "set_P_Liq.vi"("flow 1"=w316, "Run"=w315, "Bubbler In"=w317, "Active"=w317) -> ()  [unwired: 6 in]
                    }
                  }
                }
                frame #6 {
                  n292 = call "Set_Argument.vi"("Enable"=TRUE, "Argument"="run_started", "Argument List In"=w318) -> ("Argument List Out"=w319:string[])
                }
              }
            }
            frame True {
            }
          }
        }
      }
    }
    frame "End" {
    }
    frame "Idle" {
    }
  }
  "Argument List Out" <- w10
